vi "IP2 SMF in.vi"(11 "Debris out position":dbl=199.0) -> ()   [LabVIEW 2020]
panel:
  out "No errors =T 2":bool
  out "No errors =T":bool
  out "Boolean":bool
  out "Numeric 4":dbl=199.0
  in  "SMF Y in position 3":dbl=22.41
  out "Numeric 3":dbl=199.0
  in  "DPM Z in position 2":dbl=13.0
  in  "DPM X in position":dbl=107.129
  out "Numeric 2":dbl=199.0
  out "Numeric":dbl=199.0
  # "SMF In Positions"
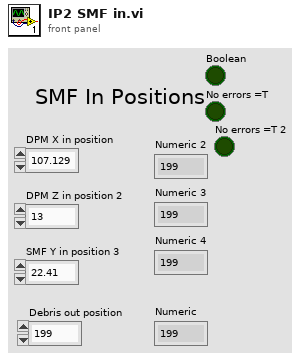
[diagram p1: front panel]
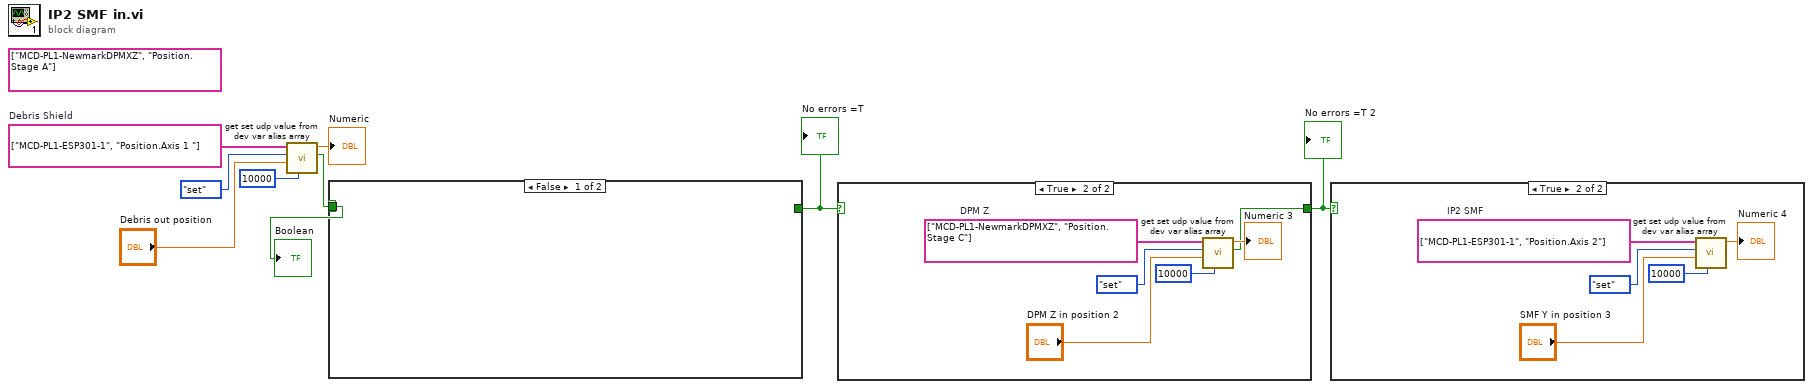
[diagram p0: block diagram]
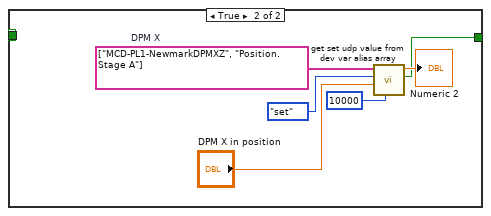
[diagram p4: hidden frame]
diagram:
  (unwired) string[] ["MCD-PL1-NewmarkDPMXZ", "Position.Stage A"] ("dev variable alias Motors X")
  w9 = string[] ["MCD-PL1-ESP301-1", "Position.Axis 1 "]  # Debris Shield
  n1 = call "get set udp value from dev var alias array.vi"("slow timeout ms (3000)"=10000, "Set position"="Debris out position", "get or set"=enum16{"get", "set"}."set", "dev variable alias Motors X"=w9) -> ("No errors =T"=w4:bool, "Numeric"=→"Numeric":dbl)  [unwired: 5 in, 1 out]
  n2 = case shown="False" w4 {
    selector: w4 -> [_ w10]
    tunnel: [_ w11] -> w3
    tunnel: [_ w10] -> w1
    frame False {
    }
    frame True {
      w16 = string[] ["MCD-PL1-NewmarkDPMXZ", "Position.Stage A"]  # DPM X
      n3 = call "get set udp value from dev var alias array.vi"("slow timeout ms (3000)"=10000, "Set position"="DPM X in position", "get or set"=enum16{"get", "set"}."set", "dev variable alias Motors X"=w16) -> ("No errors =T"=w11:bool, "Numeric"=→"Numeric 2":dbl)  [unwired: 5 in, 1 out]
    }
  }
  "Boolean" <- w1
  "No errors =T" <- w3
  n4 = case shown="True" w3 {
    tunnel: [_ w17] -> w2
    frame False {
    }
    frame True {
      w22 = string[] ["MCD-PL1-NewmarkDPMXZ", "Position.Stage C"]  # DPM Z
      n5 = call "get set udp value from dev var alias array.vi"("slow timeout ms (3000)"=10000, "Set position"="DPM Z in position 2", "get or set"=enum16{"get", "set"}."set", "dev variable alias Motors X"=w22) -> ("No errors =T"=w17:bool, "Numeric"=→"Numeric 3":dbl)  [unwired: 5 in, 1 out]
    }
  }
  "No errors =T 2" <- w2
  n6 = case shown="True" w2 {
    frame False {
    }
    frame True {
      w27 = string[] ["MCD-PL1-ESP301-1", "Position.Axis 2"]  # IP2 SMF
      n7 = call "get set udp value from dev var alias array.vi"("slow timeout ms (3000)"=10000, "Set position"="SMF Y in position 3", "get or set"=enum16{"get", "set"}."set", "dev variable alias Motors X"=w27) -> ("Numeric"=→"Numeric 4":dbl)  [unwired: 5 in, 2 out]
    }
  }
